vi "Selection.vi"   [LabVIEW 2019, in "Graph Tools.lvlib"]
doc: "Put this VI in Mouse Down Event Case for a GraphChart control"
uses:
  Graph Tools.lvlib
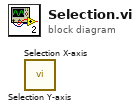
[diagram p0: block diagram]
diagram:
  n1 = call "Selection Y-axis.vi"() -> ()  [unwired: 8 in, 4 out]
  n2 = call "Selection X-axis.vi"() -> ()  [unwired: 8 in, 4 out]
